vi "Dense-Top-cell (SubVI).vi"(11 "x_dense":T1) -> (3 "y_out":T1)   [LabVIEW 2020]
uses:
  <vilib>/Analysis/Matrix/Datatypes/RealMatrix.ctl
  <vilib>/Analysis/7linalg.llb/Real Transpose Matrix.vi
  <vilib>/Analysis/Matrix/Numeric/Conversions/Array To Matrix - RA2.vi
  <vilib>/Analysis/Matrix/Numeric/Multiply/Multiply - RM,RM.vi
  <vilib>/Analysis/Matrix/Numeric/Multiply/Multiply - R,RM.vi
  <vilib>/Analysis/Matrix/NI_Matrix.lvlib
  <vilib>/Analysis/NI_AALPro.lvlib
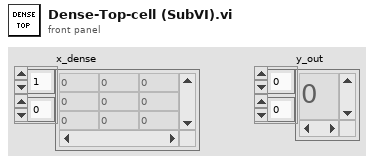
[diagram p1: front panel]
types:
  T1 = typedef "NI_Matrix.lvlib/RealMatrix.ctl" = dbl[][]
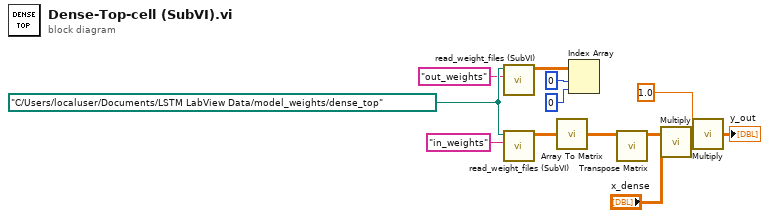
[diagram p0: block diagram]
diagram:
  w10 = path "C:/Users/localuser/Documents/LSTM LabView Data/model_weights/dense_top" ("dense top path")
  n1 = call "read_weight_files (SubVI).vi"("weight file name"="out_weights" ("String"), "weights path"=w10) -> ("all rows"=w11:dbl[][])  [unwired: 9 in]
  n2 = call "read_weight_files (SubVI).vi"("weight file name"="in_weights" ("String"), "weights path"=w10) -> ("all rows"=w8:dbl[][])  [unwired: 9 in]
  n3 = call-poly <vilib>:"Array To Matrix.vi"("Real 2D Array"=w8) -> ("Real Matrix"=w2:T1)
  n4 = Index Array(array=w11, index (row)=0, index (col)=0) -> ()  [unwired: 1 out]
  n5 = call-poly <vilib>:"Transpose Matrix.vi"("Input Matrix"=w2) -> ("Matrix Transpose"=w6:T1)  [unwired: 9 in, 1 out]
  n6 = call-poly <vilib>:"Multiply.vi"("Real Matrix B"="x_dense", "Real Matrix A"=w6) -> ("A * B"=w4:T1)
  n7 = call-poly <vilib>:"Multiply.vi"("Real Matrix A"=w4, "Real Scalar c"=1.0) -> ("c * A"=→"y_out":T1)
